vi "5.3.vi"() -> ()   [LabVIEW 2017]
panel:
  out "数组":dbl[](array[numeric])
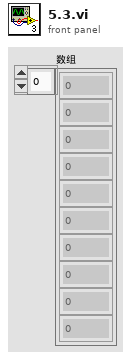
[diagram p1: front panel]
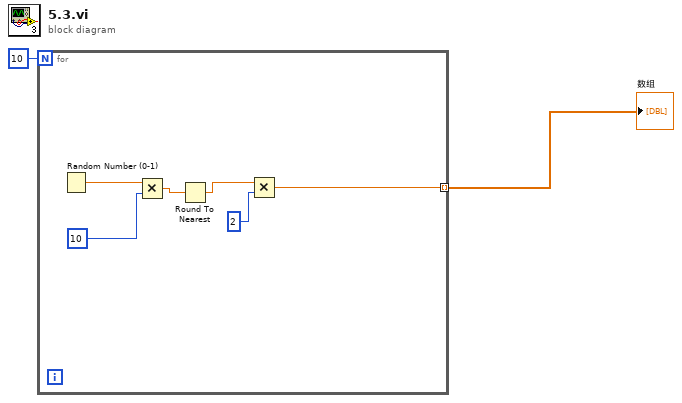
[diagram p0: block diagram]
diagram:
  n1 = for {
    N: 10 -> [_]
    tunnel: [w5] -> w1 mode=indexing
    n2 = Random Number (0-1)() -> (number: 0 to 1=w8:dbl)
    n3 = Multiply(x=w8, y=10) -> (x*y=w4:dbl)
    n4 = Round To Nearest(number=w4) -> (nearest integer value=w3:dbl)
    n5 = Multiply(x=w3, y=2) -> (x*y=w5:dbl)
  }
  "数组" <- w1
